vi "Decrement Index.vi"(8 "error in (no error)":errorcluster, 11 "Vector Parent in":refnum<class "Vector Parent.lvclass">) -> (0 "error out":errorcluster, 3 "Vector Parent out":refnum<class "Vector Parent.lvclass">)   [LabVIEW 2021, in "Vector Parent.lvclass"]
uses:
  Vector Parent.lvclass
  Vector Parent.lvclass/Vector Parent.ctl
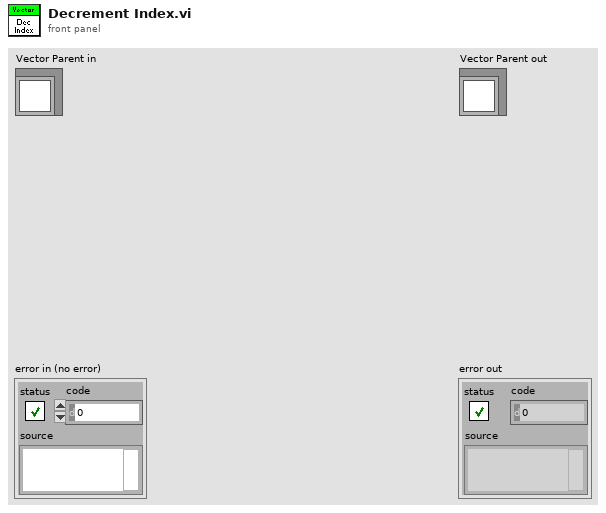
[diagram p1: front panel]
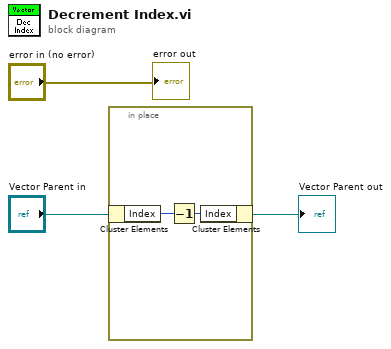
[diagram p0: block diagram]
diagram:
  n1 = in-place {
    n2 = in-place-cluster #1("Vector Parent in") -> ("Index"=w5:i32)
    n3 = Decrement(x=w5) -> (x-1=w4:i32)
    n4 = in-place-cluster #1("Index"=w4) -> (→"Vector Parent out":refnum<class "Vector Parent.lvclass">)
  }
  "error out" <- "error in (no error)"
